vi "indirect_address.vi"() -> ()   [LabVIEW 2016]
uses:
  dxl_x86_c.lvlib/dxl_x86_c.lvlib
panel:
  out "value : PRO (LED)\nmoving":bool
  in  "value : PRO (slide)\nLED RED":bool
  in  "ADDR_PRO_\nINDIRECTADDR_READ":u16=59
  in  "ADDR_PRO_\nINDIRECTADDR_WRITE":u16=49
  in  "LEN_PRO_\nINDIRECTDATA_READ":u16=5
  in  "ADDR_PRO_\nINDIRECTDATA_READ":u16=639
  in  "LEN_PRO_\nINDIRECTDATA_WRITE":u16=5
  in  "ADDR_PRO_\nINDIRECTDATA_WRITE":u16=634
  in  "LEN_PRO_\nLED_RED":u16=1
  in  "ADDR_PRO_\nLED_RED":u16=563
  in  "LEN_PRO_\nMOVING":u16=1
  in  "ADDR_PRO_\nMOVING":u16=610
  out "groupread_num":i32
  in  "LEN_PRO_\nPRESENT_POSITION":u16=4
  out "groupwrite_num":i32
  in  "LEN_PRO_\nGOAL_POSITION":u16=4
  in  "device_name":string="COM1"
  in  "ADDR_PRO_\nPRESENT_POSITION":u16=611
  in  "ADDR_PRO_\nGOAL_POSITION":u16=596
  in  "ADDR_PRO_\nTORQUE_ENABLE":u16=562
  out "protocol_version":dbl=2.0
  out "value : PRO (knob)\npresent position":i32(knob) scale=150000.0..-150000.0
  in  "terminate":bool
  out "port_num":i32
  in  "value : PRO (dial)\ngoal position":i32(knob) scale=150000.0..-150000.0
  in  "dynamixel_id":u8=1
  in  "baud_rate":i32=1000000
  # "/*******************************************************************************\n* Copyright (c) 2016, ROBOTIS CO., LTD.\n* All rights reserved.\n*\n* Redistribution and use in source and binary forms, with or without\n* modification, are permitted provided that the following conditions are met:\n*\n* * Redistributions of source code must retain the above copyright notice, this\n*   list of conditions and the following disclaimer.\n*\n* * Redistributions in binary form must reproduce the above copyright notice,\n*   this list of conditions and the following disclaimer in the documentation\n*   and/or other materials provided with the distribution.\n*\n* * Neither the name of ROBOTIS nor the names of its\n*   contributors may be used to endorse or promote products derived from\n*   this software without specific prior written permission.\n*\n* THIS SOFTWARE IS PROVIDED BY THE COPYRIGHT HOLDERS AND CONTRIBUTORS \"AS IS\"\n* AND ANY EXPRESS OR IMPLIED WARRANTIES, INCLUDING, BUT NOT LIMITED TO, THE\n* IMPLIED WARRANTIES OF MERCHANTABILITY AND FITNESS FOR A PARTICULAR PURPOSE ARE\n* DISCLAIMED. IN NO EVENT SHALL THE COPYRIGHT HOLDER OR CONTRIBUTORS BE LIABLE\n* FOR ANY DIRECT, INDIRECT, INCIDENTAL, SPECIAL, EXEMPLARY, OR CONSEQUENTIAL\n* DAMAGES (INCLUDING, BUT NOT LIMITED TO, PROCUREMENT OF SUBSTITUTE GOODS OR\n* SERVICES; LOSS OF USE, DATA, OR PROFITS; OR BUSINESS INTERRUPTION) HOWEVER\n* CAUSED AND ON ANY THEORY OF LIABILITY, WHETHER IN CONTRACT, STRICT LIABILITY,\n* OR TORT (INCLUDING NEGLIGENCE OR OTHERWISE) ARISING IN ANY WAY OUT OF THE USE\n* OF THIS SOFTWARE, EVEN IF ADVISED OF THE POSSIBILITY OF SUCH DAMAGE.\n*******************************************************************************/\n\n/* Author: Ryu Woon Jung (Leon) */"
  # "Available Dynamixel model on this example : All models using Protocol 2.0\nThis example is designed for using a Dynamixel PRO 54-200, and an USB2DYNAMIXEL.\nTo use another Dynamixel model, such as X series, see their details in E-Manual(support.robotis.com) \n   and edit \"numeric control\"s seen left with \"Edit Text\" tool.\nBe sure that Dynamixel PRO properties are already set as %% ID : 1 / Baudnum : 1 (Baudrate : 57600)\n\n1. Run example by click above \"Run\" button (below \"Edit\" menu).\n2. Drag \"dial\" then you may see the Dynamixel and \"knob\"s rotating\n3. Click \"slide button\" then you may see the LED of Dynamixel lighting\n4. To finish the example, press \"terminate\" button."
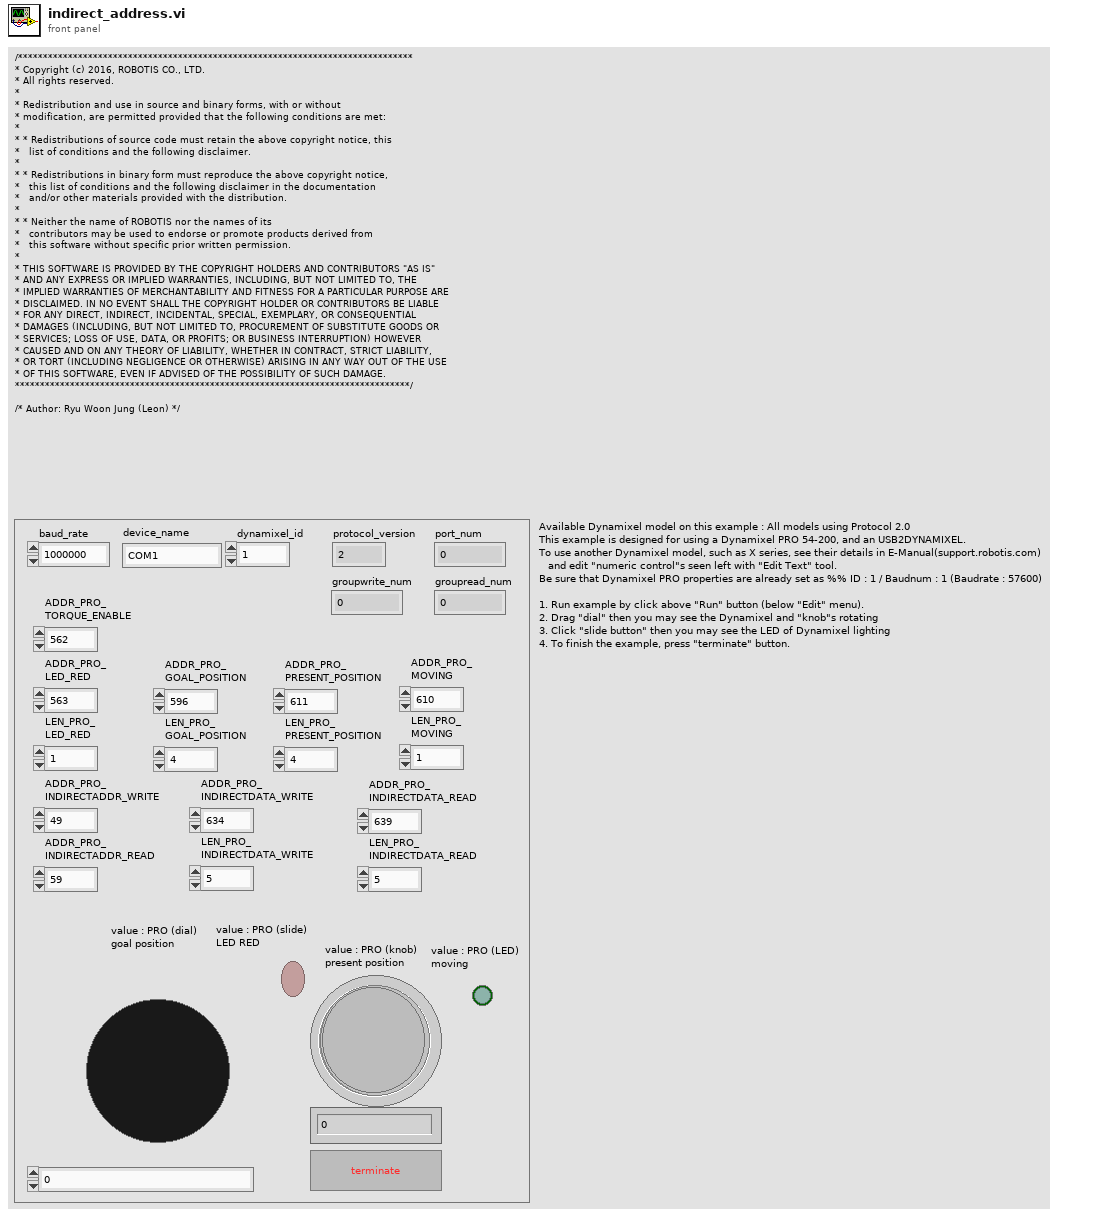
[diagram p1: front panel]
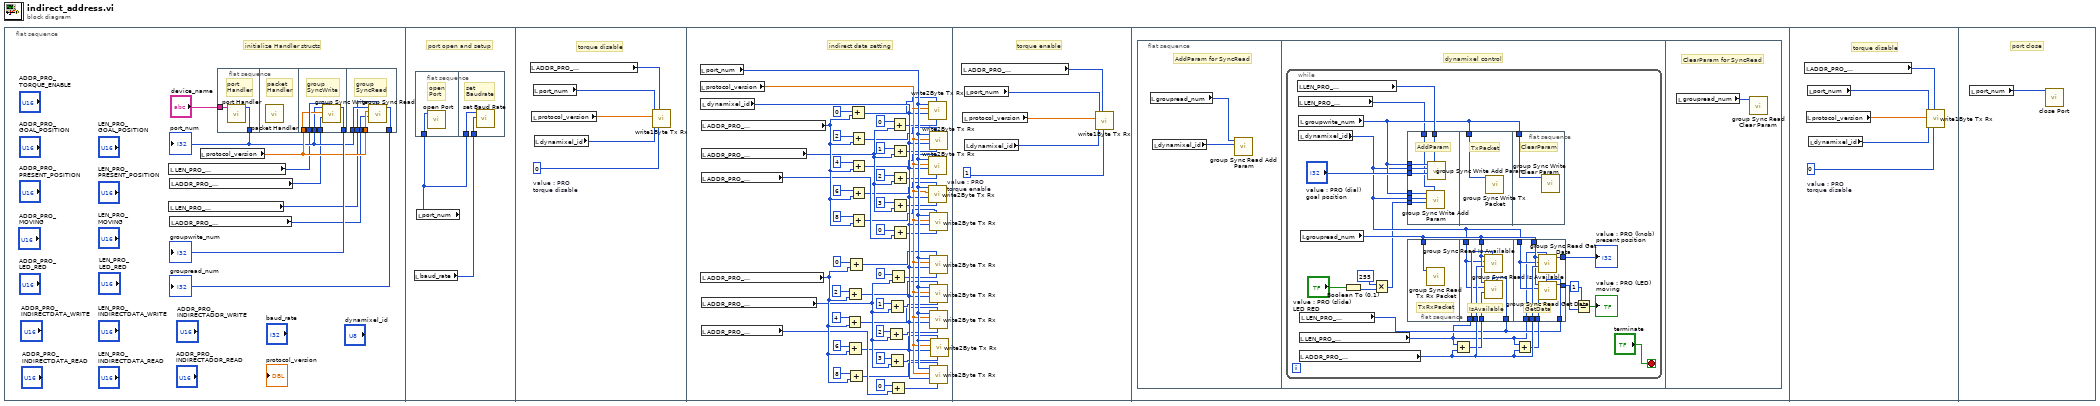
[diagram p0: block diagram]
diagram:
  n1 = flat-sequence {
    frame #0 {
      # "initialize Handler structs"
      n2 = local read "LEN_PRO_\nINDIRECTDATA_WRITE"() -> (w1:u16)
      n3 = local read "LEN_PRO_\nINDIRECTDATA_READ"() -> (w3:u16)
      n4 = local read "ADDR_PRO_\nINDIRECTDATA_WRITE"() -> (w2:u16)
      n5 = local read "ADDR_PRO_\nINDIRECTDATA_READ"() -> (w4:u16)
      n6 = local read "protocol_version"() -> (w6:dbl)
      n7 = flat-sequence {
        tunnel: "device_name" -> [w11]
        tunnel: [w10] -> w5
        tunnel: w1 -> [w16]
        tunnel: w2 -> [w15]
        tunnel: w6 -> [w14]
        tunnel: w5 -> [w13]
        tunnel: [w12] -> w8
        tunnel: [w21] -> w7
        tunnel: w6 -> [w20]
        tunnel: w4 -> [w19]
        tunnel: w5 -> [w18]
        tunnel: w3 -> [w17]
        frame #0 {
          # "port\nHandler"
          n8 = call "port Handler.vi"("port_name"=w11) -> ("function return"=w10:i32)  [unwired: 10 in]
        }
        frame #1 {
          # "packet\nHandler"
          n9 = call "packet Handler.vi"() -> ()  [unwired: 12 in]
        }
        frame #2 {
          # "group\nSyncWrite"
          n10 = call "group Sync Write.vi"("data_length"=w16, "start_address"=w15, "protocol_version"=w14, "port_num"=w13) -> ("function return"=w12:i32)  [unwired: 7 in]
        }
        frame #3 {
          # "group\nSyncRead"
          n11 = call "group Sync Read.vi"("data_length"=w17, "start_address"=w19, "protocol_version"=w20, "port_num"=w18) -> ("function return"=w21:i32)  [unwired: 7 in]
        }
      }
      "port_num" <- w5
      "groupwrite_num" <- w8
      "groupread_num" <- w7
    }
    frame #1 {
      # "port open and setup"
      n12 = local read "baud_rate"() -> (w22:i32)
      n13 = flat-sequence {
        tunnel: w23 -> [w24]
        tunnel: w23 -> [w26]
        tunnel: w22 -> [w25]
        frame #0 {
          # "open\nPort"
          n14 = call "open Port.vi"("port_num"=w24) -> ()  [unwired: 10 in, 1 out]
        }
        frame #1 {
          # "set\nBaudrate"
          n15 = call "set Baud Rate.vi"("baudrate"=w25, "port_num"=w26) -> ()  [unwired: 9 in, 1 out]
        }
      }
      n16 = local read "port_num"() -> (w23:i32)
    }
    frame #2 {
      w30 = 0  # value : PRO torque disable
      # "torque disable"
      n17 = local read "ADDR_PRO_\nTORQUE_ENABLE"() -> (w28:u16)
      n18 = local read "protocol_version"() -> (w29:dbl)
      n19 = local read "port_num"() -> (w31:i32)
      n20 = local read "dynamixel_id"() -> (w27:u8)
      n21 = call "write1Byte Tx Rx.vi"("data"=w30, "address"=w28, "id"=w27, "protocol_version"=w29, "port_num"=w31) -> ()  [unwired: 7 in]
    }
    frame #3 {
      # "indirect data setting"
      n22 = local read "port_num"() -> (w54:i32)
      n23 = local read "protocol_version"() -> (w53:dbl)
      n24 = local read "dynamixel_id"() -> (w52:u8)
      n25 = local read "ADDR_PRO_\nINDIRECTADDR_READ"() -> (w59:u16)
      n26 = local read "ADDR_PRO_\nINDIRECTADDR_WRITE"() -> (w60:u16)
      n27 = local read "ADDR_PRO_\nGOAL_POSITION"() -> (w58:u16)
      n28 = local read "ADDR_PRO_\nLED_RED"() -> (w57:u16)
      n29 = local read "ADDR_PRO_\nPRESENT_POSITION"() -> (w56:u16)
      n30 = local read "ADDR_PRO_\nMOVING"() -> (w55:u16)
      n31 = Add(x=4, y=w59) -> (x+y=w39:i32)
      n32 = Add(x=2, y=w59) -> (x+y=w40:i32)
      n33 = Add(x=6, y=w59) -> (x+y=w38:i32)
      n34 = Add(x=0, y=w59) -> (x+y=w41:i32)
      n35 = Add(x=8, y=w59) -> (x+y=w37:i32)
      n36 = Add(x=0, y=w60) -> (x+y=w46:i32)
      n37 = Add(x=2, y=w60) -> (x+y=w45:i32)
      n38 = Add(x=4, y=w60) -> (x+y=w44:i32)
      n39 = Add(x=6, y=w60) -> (x+y=w43:i32)
      n40 = Add(x=8, y=w60) -> (x+y=w42:i32)
      n41 = Add(x=2, y=w56) -> (x+y=w49:i32)
      n42 = Add(x=1, y=w56) -> (x+y=w48:i32)
      n43 = Add(x=3, y=w56) -> (x+y=w50:i32)
      n44 = Add(x=0, y=w56) -> (x+y=w47:i32)
      n45 = Add(x=0, y=w55) -> (x+y=w51:i32)
      n46 = Add(x=0, y=w58) -> (x+y=w32:i32)
      n47 = Add(x=1, y=w58) -> (x+y=w33:i32)
      n48 = Add(x=2, y=w58) -> (x+y=w34:i32)
      n49 = Add(x=3, y=w58) -> (x+y=w35:i32)
      n50 = Add(x=0, y=w57) -> (x+y=w36:i32)
      n51 = call "write2Byte Tx Rx.vi"("data"=w32, "address"=w46, "id"=w52, "protocol_version"=w53, "port_num"=w54) -> ()  [unwired: 7 in]
      n52 = call "write2Byte Tx Rx.vi"("data"=w34, "address"=w44, "id"=w52, "protocol_version"=w53, "port_num"=w54) -> ()  [unwired: 7 in]
      n53 = call "write2Byte Tx Rx.vi"("data"=w35, "address"=w43, "id"=w52, "protocol_version"=w53, "port_num"=w54) -> ()  [unwired: 7 in]
      n54 = call "write2Byte Tx Rx.vi"("data"=w33, "address"=w45, "id"=w52, "protocol_version"=w53, "port_num"=w54) -> ()  [unwired: 7 in]
      n55 = call "write2Byte Tx Rx.vi"("data"=w36, "address"=w42, "id"=w52, "protocol_version"=w53, "port_num"=w54) -> ()  [unwired: 7 in]
      n56 = call "write2Byte Tx Rx.vi"("data"=w47, "address"=w41, "id"=w52, "protocol_version"=w53, "port_num"=w54) -> ()  [unwired: 7 in]
      n57 = call "write2Byte Tx Rx.vi"("data"=w48, "address"=w40, "id"=w52, "protocol_version"=w53, "port_num"=w54) -> ()  [unwired: 7 in]
      n58 = call "write2Byte Tx Rx.vi"("data"=w49, "address"=w39, "id"=w52, "protocol_version"=w53, "port_num"=w54) -> ()  [unwired: 7 in]
      n59 = call "write2Byte Tx Rx.vi"("data"=w51, "address"=w37, "id"=w52, "protocol_version"=w53, "port_num"=w54) -> ()  [unwired: 7 in]
      n60 = call "write2Byte Tx Rx.vi"("data"=w50, "address"=w38, "id"=w52, "protocol_version"=w53, "port_num"=w54) -> ()  [unwired: 7 in]
    }
    frame #4 {
      w82 = 1  # value : PRO torque enable
      # "torque enable"
      n61 = local read "ADDR_PRO_\nTORQUE_ENABLE"() -> (w84:u16)
      n62 = local read "protocol_version"() -> (w83:dbl)
      n63 = local read "port_num"() -> (w81:i32)
      n64 = local read "dynamixel_id"() -> (w85:u8)
      n65 = call "write1Byte Tx Rx.vi"("data"=w82, "address"=w84, "id"=w85, "protocol_version"=w83, "port_num"=w81) -> ()  [unwired: 7 in]
    }
    frame #5 {
      n66 = flat-sequence {
        frame #0 {
          # "AddParam for SyncRead"
          n67 = local read "groupread_num"() -> (w86:i32)
          n68 = local read "dynamixel_id"() -> (w87:u8)
          n69 = call "group Sync Read Add Param.vi"("id"=w87, "group_num"=w86) -> ()  [unwired: 9 in, 1 out]
        }
        frame #1 {
          # "dynamixel control"
          n70 = while {
            stop <- "terminate" stop-if-true
            n71 = local read "LEN_PRO_\nGOAL_POSITION"() -> (w106:u16)
            n72 = local read "LEN_PRO_\nLED_RED"() -> (w96:u16)
            n73 = local read "groupwrite_num"() -> (w102:i32)
            n74 = local read "dynamixel_id"() -> (w101:u8)
            n75 = local read "LEN_PRO_\nPRESENT_POSITION"() -> (w88:u16)
            n76 = local read "ADDR_PRO_\nINDIRECTDATA_READ"() -> (w95:u16)
            n77 = local read "LEN_PRO_\nMOVING"() -> (w89:u16)
            n78 = local read "groupread_num"() -> (w104:i32)
            n79 = Boolean To (0,1)(Boolean="value : PRO (slide)\nLED RED") -> (0, 1=w99:i16)
            n80 = Multiply(x=255, y=w99) -> (x*y=w97:i32)
            n81 = flat-sequence {
              tunnel: w106 -> [w130]
              tunnel: w102 -> [w129]
              tunnel: w101 -> [w128]
              tunnel: "value : PRO (dial)\ngoal position" -> [w127]
              tunnel: w102 -> [w126]
              tunnel: w101 -> [w125]
              tunnel: w97 -> [w124]
              tunnel: w96 -> [w123]
              tunnel: w102 -> [w131]
              tunnel: w102 -> [w132]
              frame #0 {
                # "AddParam"
                n82 = call "group Sync Write Add Param.vi"("data_length"=w123, "data"=w124, "id"=w125, "group_num"=w126) -> ()  [unwired: 7 in, 1 out]
                n83 = call "group Sync Write Add Param.vi"("data_length"=w130, "data"=w127, "id"=w128, "group_num"=w129) -> ()  [unwired: 7 in, 1 out]
              }
              frame #1 {
                # "TxPacket"
                n84 = call "group Sync Write Tx Packet.vi"("group_num"=w131) -> ()  [unwired: 11 in]
              }
              frame #2 {
                # "ClearParam"
                n85 = call "group Sync Write Clear Param.vi"("group_num"=w132) -> ()  [unwired: 11 in]
              }
            }
            n86 = flat-sequence {
              tunnel: w104 -> [w108]
              tunnel: w104 -> [w112]
              tunnel: w101 -> [w111]
              tunnel: w95 -> [w114]
              tunnel: w88 -> [w113]
              tunnel: w94 -> [w110]
              tunnel: w89 -> [w109]
              tunnel: w104 -> [w120]
              tunnel: w101 -> [w119]
              tunnel: [w122] -> w103
              tunnel: w95 -> [w121]
              tunnel: w93 -> [w118]
              tunnel: w89 -> [w117]
              tunnel: [w116] -> w90
              tunnel: w88 -> [w115]
              frame #0 {
                # "TxRxPacket"
                n87 = call "group Sync Read Tx Rx Packet.vi"("group_num"=w108) -> ()  [unwired: 11 in]
              }
              frame #1 {
                # "IsAvailable"
                n88 = call "group Sync Read Is Available.vi"("data_length"=w113, "address"=w114, "id"=w111, "group_num"=w112) -> ()  [unwired: 7 in, 1 out]
                n89 = call "group Sync Read Is Available.vi"("data_length"=w109, "address"=w110, "id"=w111, "group_num"=w112) -> ()  [unwired: 7 in, 1 out]
              }
              frame #2 {
                # "GetData"
                n90 = call "group Sync Read Get Data.vi"("data_length"=w115, "address"=w121, "id"=w119, "group_num"=w120) -> ("function return"=w122:u32)  [unwired: 7 in]
                n91 = call "group Sync Read Get Data.vi"("data_length"=w117, "address"=w118, "id"=w119, "group_num"=w120) -> ("function return"=w116:u32)  [unwired: 7 in]
              }
            }
            n92 = Add(x=w88, y=w95) -> (x+y=w94:u16)
            n93 = Add(x=w88, y=w95) -> (x+y=w93:u16)
            n94 = Equal?(x=1, y=w90) -> (x = y?=→"value : PRO (LED)\nmoving":bool)
            "value : PRO (knob)\npresent position" <- w103
          }
        }
        frame #2 {
          # "ClearParam for SyncRead"
          n95 = local read "groupread_num"() -> (w133:i32)
          n96 = call "group Sync Read Clear Param.vi"("group_num"=w133) -> ()  [unwired: 11 in]
        }
      }
    }
    frame #6 {
      w135 = 0  # value : PRO torque disable
      # "torque disable"
      n97 = local read "ADDR_PRO_\nTORQUE_ENABLE"() -> (w137:u16)
      n98 = local read "protocol_version"() -> (w136:dbl)
      n99 = local read "port_num"() -> (w134:i32)
      n100 = local read "dynamixel_id"() -> (w138:u8)
      n101 = call "write1Byte Tx Rx.vi"("data"=w135, "address"=w137, "id"=w138, "protocol_version"=w136, "port_num"=w134) -> ()  [unwired: 7 in]
    }
    frame #7 {
      # "port close"
      n102 = local read "port_num"() -> (w139:i32)
      n103 = call "close Port.vi"("port_num"=w139) -> ()  [unwired: 11 in]
    }
  }
